vi "update progress bar.vi"(3 "Hold Stage":bool, 6 "Max":i32, 7 "Progress":i32) -> (1 "Write progress":u8(slide) scale=0.0..100.0)   [LabVIEW 2018]
uses:
  CAEN globals.vi
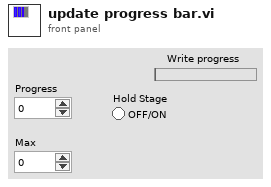
[diagram p1: front panel]
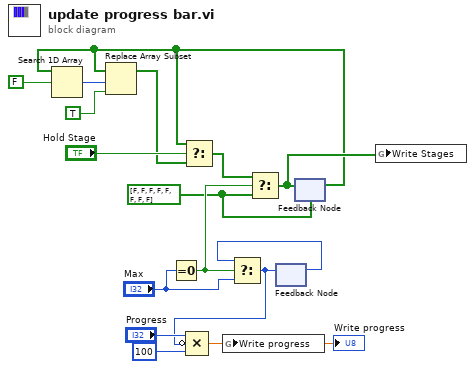
[diagram p0: block diagram]
diagram:
  w6 = bool[] [FALSE, FALSE, FALSE, FALSE, FALSE, FALSE, FALSE, FALSE] ("Write Stages")
  n1 = Equal To 0?(x="Max") -> (x = 0?=w10:bool)
  n2 = feedback #1() -> (w12:i32)  [unwired: 1 in]
  n3 = Select(t=w12, s=w10, f="Max") -> (s? t:f=w14:i32)
  n4 = Compound Arithmetic op=MULTIPLY("Progress", invert w14, 100 ("value")) -> (w11:dbl)
  "Write progress" <- w11
  n5 = global write "CAEN globals.vi" "Write progress"(w11) -> ()
  n6 = feedback-in #1(w14) -> ()
  n7 = feedback #2(w6) -> (w1:bool[])
  n8 = Search 1D Array(1D array=w1, element=FALSE) -> (index of element=w8:i32)  [unwired: 1 in]
  n9 = Replace Array Subset(array=w1, new element=TRUE, index=w8) -> (w2:bool[])
  n10 = Select(t=w1, s="Hold Stage", f=w2) -> (s? t:f=w4:bool[])
  n11 = Select(t=w4, s=w10, f=w6) -> (s? t:f=w5:bool[])
  n12 = feedback-in #2(w5) -> ()
  n13 = global write "CAEN globals.vi" "Write Stages"(w5) -> ()
